vi "errorNumberToRecommendation.vi"(8 "error in":errorcluster, 9 "errNbr":i32, 10 "language":i32, 11 "connection ID":i32) -> (0 "error out":errorcluster, 2 "string":string, 3 "connection ID":i32)   [LabVIEW 2016]
doc: "Get a recommendation for the error code"
panel:
  out "params_cluster":cluster{"language":i32, "errNbr":i32}
  in  "Params_cluster":cluster{"integer":i32, "integer":i32}
  in  "results_cluster":cluster{"errNo":i32, "string":string}
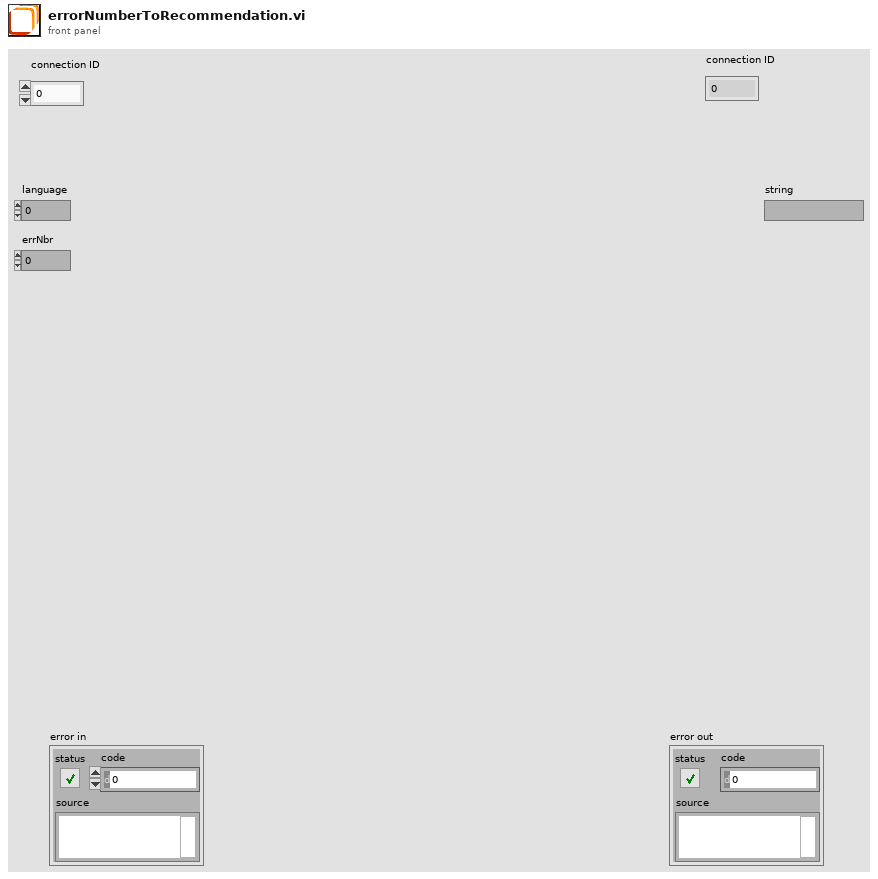
[diagram p1: front panel]
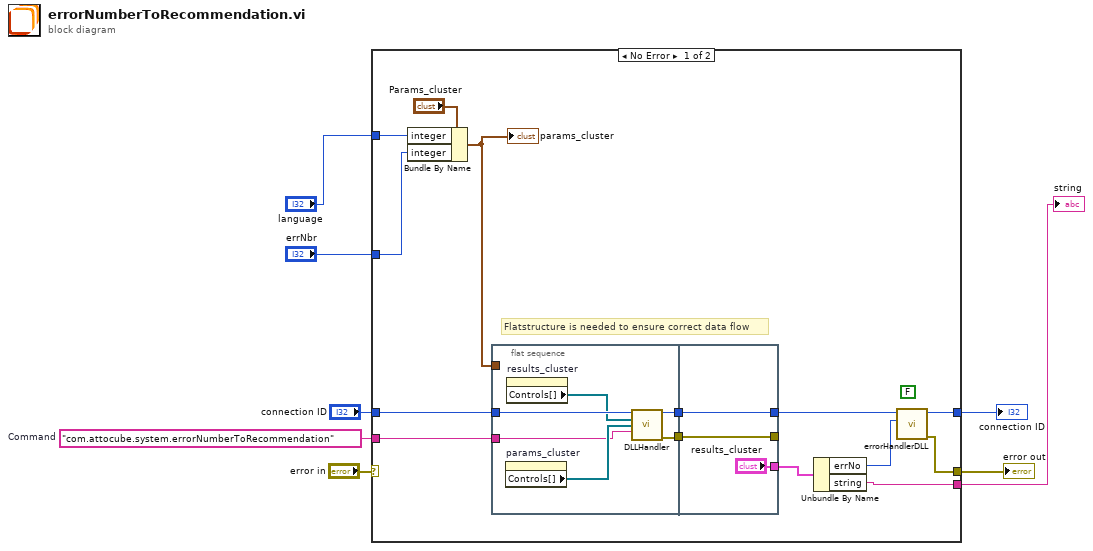
[diagram p0: block diagram]
diagram:
  w6 = "com.attocube.system.errorNumberToRecommendation"  # Command
  n1 = case shown="No Error" "error in" {
    selector: "error in" -> [_ w33]
    tunnel: [w12 w33] -> w8
    tunnel: "connection ID" -> [w22 w32]
    tunnel: w6 -> [w19 _]
    tunnel: [w14 w32] -> w4
    tunnel: "language" -> [w11 _]
    tunnel: "errNbr" -> [w10 _]
    tunnel: [w9 _] -> w1
    frame No Error {
      (unwired) FALSE ("show popup")
      # "Flatstructure is needed to ensure correct data flow"
      n2 = Bundle By Name(cluster="Params_cluster", "integer"=w11, "integer"=w10) -> (w17:cluster{"integer":i32, "integer":i32})
      "params_cluster" <- w17
      n3 = flat-sequence {
        tunnel: w22 -> [w28]
        tunnel: w19 -> [w25]
        tunnel: [w24] -> w18
        tunnel: w17 -> [_]
        tunnel: [w23] -> w15
        tunnel: ["results_cluster"] -> w21
        tunnel: [w31] -> w16
        tunnel: [w29] -> _
        tunnel: w18 -> [w29]
        tunnel: w15 -> [w31]
        frame #0 {
          n4 = property on="params_cluster" class="Clust (strict)"() -> ("Controls[]"=w26:refnum<vi>[])  [unwired: 2 in, 2 out]
          n5 = property on="results_cluster" class="Clust (strict)"() -> ("Controls[]"=w27:refnum<vi>[])  [unwired: 2 in, 2 out]
          n6 = call "DLLHandler.vi"("connection ID"=w28, "results_cluster"=w27, "params_cluster"=w26, "method"=w25) -> ("connection ID out"=w23:i32, "error"=w24:errorcluster)  [unwired: 10 in]
        }
        frame #1 {
        }
      }
      n7 = Unbundle By Name(w21) -> ("errNo"=w13:i32, "string"=w9:string)
      n8 = call "errorHandlerDLL.vi"("error number"=w13, "connection ID"=w16) -> ("error out"=w12:errorcluster, "connection ID"=w14:i32)  [unwired: 8 in]
    }
    frame Error {
    }
  }
  "error out" <- w8
  "connection ID" <- w4
  "string" <- w1
